vi "Update Layout.vi"(8 "error in (no error)":errorcluster, 11 "PanelArray in":refnum<class "PanelArray.lvclass">) -> (0 "error out":errorcluster, 3 "PanelArray out":refnum<class "PanelArray.lvclass">)   [LabVIEW 2018, in "OOPanel.lvlib" / "PanelArray.lvclass"]
uses:
  PanelArray.lvclass
  PanelArray.lvclass/PanelArray.ctl
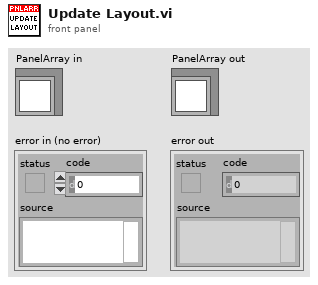
[diagram p1: front panel]
types:
  T1 = typedef "OOPanel.lvlib/PanelArray.lvclass/Ref Data.ctl" = cluster{"State":T2, "Refs":T3, "Events":T4, "Scrolling":T5, "Panels":T6}
  T2 = typedef "OOPanel.lvlib/PanelArray.lvclass/State.ctl" = cluster{"Defer Updates":bool, "Running":bool, "Dynamic Sizing":bool, "Borders":bool}
  T3 = typedef "OOPanel.lvlib/PanelArray.lvclass/Refs.ctl" = cluster{"SubPanels":refnum<vi>[], "Scrollbar":refnum<vi>, "Owning Panel":refnum<vi>}
  T4 = typedef "OOPanel.lvlib/PanelArray.lvclass/Events.ctl" = cluster{"Close":refnum<user-event>}
  T5 = typedef "OOPanel.lvlib/PanelArray.lvclass/Scrolling.ctl" = cluster{"Size":i32, "Max":i32, "Current":i32, "Top Index":i32, "Heights":i32[]}
  T6 = typedef "OOPanel.lvlib/PanelArray.lvclass/Panels.ctl" = cluster{"All":refnum<class "Panel.lvclass">[], "Visible":refnum<class "Panel.lvclass">[], "Blank":refnum<class "ArrayBlank.lvclass">}
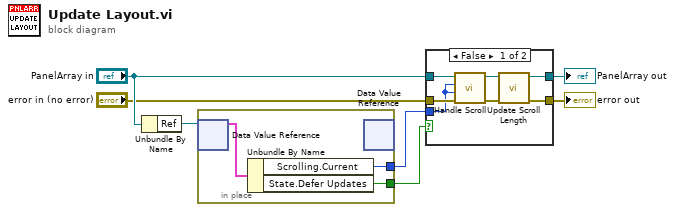
[diagram p0: block diagram]
diagram:
  n1 = Unbundle By Name("PanelArray in") -> ("Ref"=w7:refnum<data-value>)
  n2 = in-place {
    in-place-border: [w9] -> w2
    in-place-border: [w8] -> w1
    n3 = in-place-dvr #1(w7) -> (w10:T1)  [unwired: 1 out]
    n4 = Unbundle By Name(w10) -> ("Scrolling.Current"=w9:i32, "State.Defer Updates"=w8:bool)
    n5 = in-place-dvr #1() -> ()  [unwired: 1 in, 2 out]
  }
  n6 = case shown="False" w1 {
    tunnel: "PanelArray in" -> [w17 w19]
    tunnel: [w12 w19] -> w5
    tunnel: [w11 w18] -> w4
    tunnel: "error in (no error)" -> [w16 w18]
    tunnel: w2 -> [w15 _]
    frame False {
      n7 = call "Handle Scroll.vi"("error in (no error)"=w16, "OldVal"=w15, "NewVal"=w15, "PanelArray in"=w17) -> ("error out"=w14:errorcluster, "PanelArray out"=w13:refnum<class "PanelArray.lvclass">)  [unwired: 6 in]
      n8 = call "Update Scroll Length.vi"("error in (no error)"=w14, "PanelArray in"=w13) -> ("error out"=w11:errorcluster, "PanelArray out"=w12:refnum<class "PanelArray.lvclass">)  [unwired: 8 in]
    }
    frame True {
    }
  }
  "error out" <- w4
  "PanelArray out" <- w5
